vi "Loop_Overlord.vi"() -> ()   [LabVIEW 2017, in "Rotation_Overlord.lvlib"]
uses:
  Rotation_Overlord.lvlib
  _SHARE ALL/Global Share All/Global_STOP.vi
  ENUM_Overloard_Action.ctl
  ENUM_Overloard_State.ctl
  Arm/ENUM_SM_Rotate_Positions.ctl
  Arm/Arm.lvlib
  Arm/CLUSTER_CMD_SM_Lift_Rotate.ctl
  Claw Rotation/ENUM_SM_Rotate_Positions.ctl
  Claw Rotation/Claw_Rotation.lvlib
  Claw Rotation/CLUSTER_CMD_SM_Lift_Rotate.ctl
  Lift/ENUM_SM_Rotate_Positions.ctl
  Lift/Lift.lvlib
  Lift/CLUSTER_CMD_SM_Lift_Rotate.ctl
  Arm/Global_CMD.vi
  Claw Rotation/Global_CMD.vi
  Lift/Global_CMD.vi
  ENUM_Rotation_Positon.ctl
  CLUSTER_Rotation_CMD.ctl
  Global_CMD.vi
  Arm/ENUM_SM_State.ctl
  Claw Rotation/ENUM_SM_State.ctl
  Lift/ENUM_SM_State.ctl
  Arm/Global_SM Write_Data Out.vi
  Claw Rotation/Global_SM Write_Data Out.vi
  Lift/Global_SM Write_Data Out.vi
panel:
  out "Input DBL Data":dbl
  out "Output Bool Data":bool
  out "Output DBL Data":dbl
  out "OutputI INT Data":i32
  out "Cycle Time (S)":dbl format="%.3g"
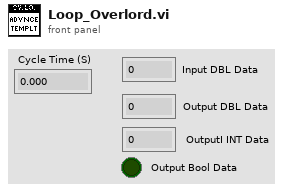
[diagram p1: front panel]
types:
  T1 = typedef "Lift.lvlib/ENUM_SM_State.ctl" = enum16{"Startup", "Idle", "Manual", "Position - Moving", "Position - Holding", "Shutdown"}
  T2 = typedef "Claw_Rotation.lvlib/ENUM_SM_State.ctl" = enum16{"Startup", "Idle", "Manual", "Position - Moving", "Position - Holding", "Shutdown"}
  T3 = typedef "Arm.lvlib/ENUM_SM_State.ctl" = enum16{"Startup", "Idle", "Manual", "Position - Moving", "Position - Holding", "Shutdown"}
  T4 = typedef "Rotation_Overlord.lvlib/CLUSTER_Rotation_CMD.ctl" = cluster{"Rotation Positon":T5, "Enable Rotation":bool}
  T5 = typedef "Rotation_Overlord.lvlib/ENUM_Rotation_Positon.ctl" = enum16{"Neutral", "Pickup", "Exchange", "Switch", "Scale", "Climb", "Manual"}
  T6 = typedef "Lift.lvlib/CLUSTER_CMD_SM_Lift_Rotate.ctl" = cluster{"Enable System":bool, "Rotate Position":T7, "Manual Velocity":dbl, "Manual Mode":bool}
  T7 = typedef "Lift.lvlib/ENUM_SM_Rotate_Positions.ctl" = enum16{"Neutral: 0", "Pickup: 0", "Exchange: 0", "Switch: 0", "Scale: 0", "Climb: 0"}
  T8 = typedef "Claw_Rotation.lvlib/CLUSTER_CMD_SM_Lift_Rotate.ctl" = cluster{"Enable System":bool, "Rotate Position":T9, "Manual Velocity":dbl, "Manual Mode":bool}
  T9 = typedef "Claw_Rotation.lvlib/ENUM_SM_Rotate_Positions.ctl" = enum16{"Neutral: 0", "Pickup: 0", "Exchange: 0", "Switch: 0", "Scale: 0", "Climb: 0"}
  T10 = typedef "Arm.lvlib/CLUSTER_CMD_SM_Lift_Rotate.ctl" = cluster{"Enable System":bool, "Rotate Position":T11, "Manual Velocity":dbl, "Manual Mode":bool}
  T11 = typedef "Arm.lvlib/ENUM_SM_Rotate_Positions.ctl" = enum16{"Neutral: 0", "Pickup: 0", "Exchange: 0", "Switch: 0", "Scale: 0", "Climb: 0"}
  T12 = typedef "Rotation_Overlord.lvlib/ENUM_Overloard_State.ctl" = enum16{"Startup", "Idle", "Neutral - Moving", "Neutral - Holding", "Pickup - Moving", "Pickup - Holding", "Exchange - Moving", "Exchange - Holding", "Switch - Moving", "Switch - Holding", "Scale - Moving", "Scale - Holding", "Climb - Moving", "Climb - Holding", "Manual", "Shutdown"}
  T13 = typedef "Rotation_Overlord.lvlib/ENUM_Overloard_Action.ctl" = enum16{"No Action", "Reset Time", "Disable All", "Disable Lift", "Disable Arm", "Disable Claw Rotation", "Set Neutral", "Set Pickup", "Set Exchange", "Set Switch", "Set Scale", "Set Climb", "Manual"}
  T14 = cluster{"State":T12, "Previous State":T12, "Current Time":timestamp, "Previous Time":timestamp, "Start Time":timestamp, "Target Time (ms)":u32, "Cycle Time(S)":dbl, "Arm CMD":T10, "Claw Rotation CMD":T8, "Lift CMD":T6, "Rotation CMD":T4, "Arm State":T3, "Claw Rotation State":T2, "Lift State":T1}
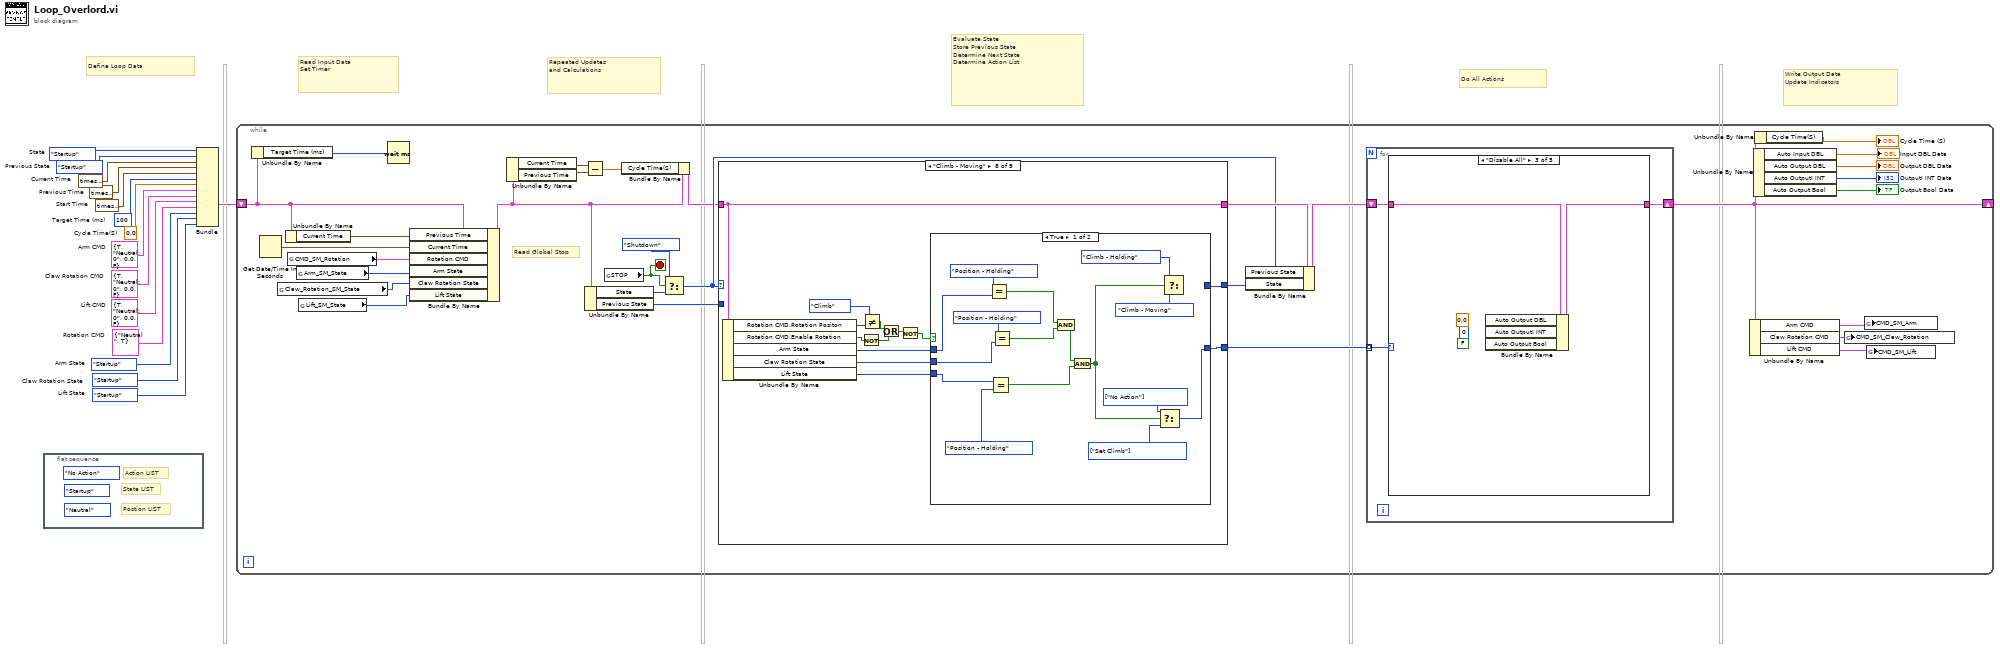
[diagram p0: block diagram]
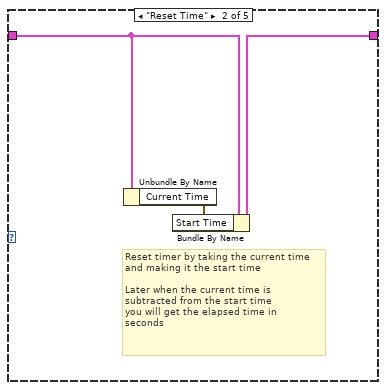
[diagram p3: hidden frame]
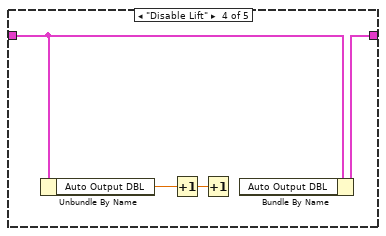
[diagram p4: hidden frame]
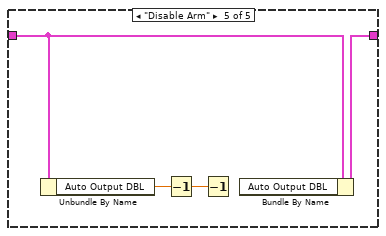
[diagram p5: hidden frame]
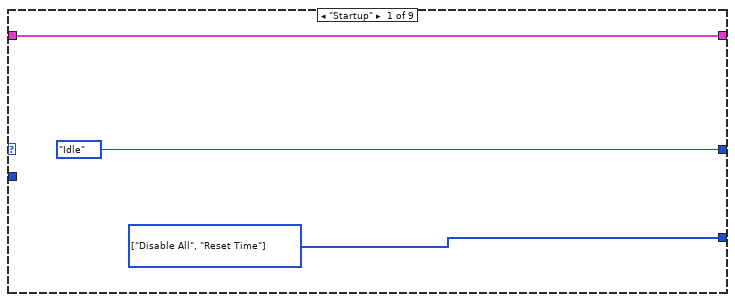
[diagram p6: hidden frame]
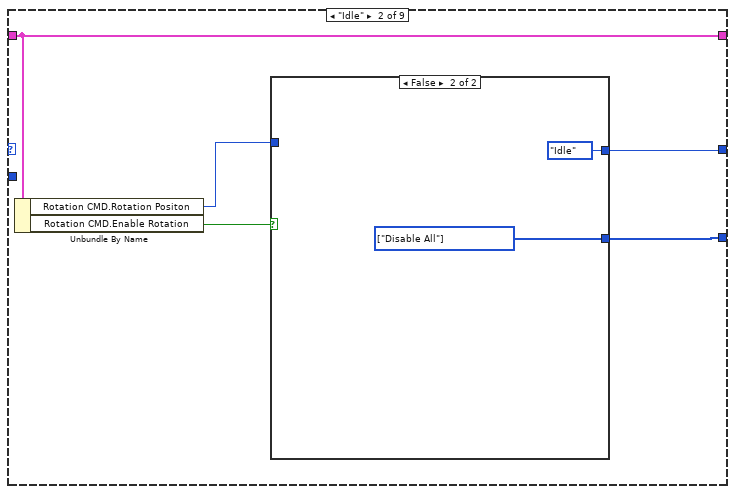
[diagram p7: hidden frame]
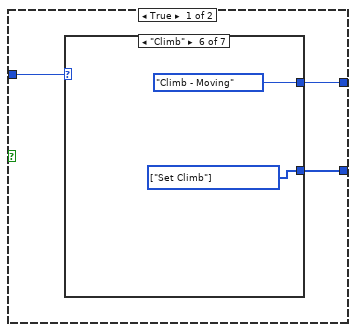
[diagram p8: hidden frame]
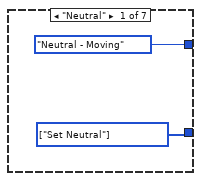
[diagram p9: hidden frame]
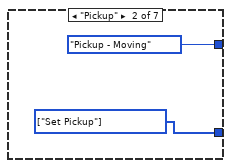
[diagram p10: hidden frame]
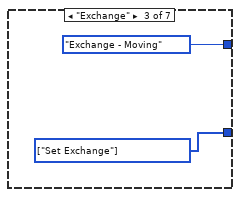
[diagram p11: hidden frame]
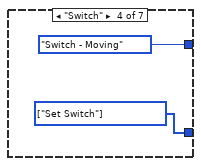
[diagram p12: hidden frame]
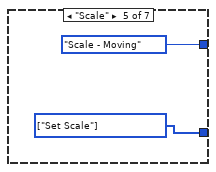
[diagram p13: hidden frame]
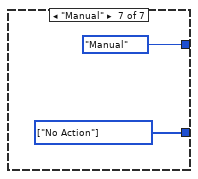
[diagram p14: hidden frame]
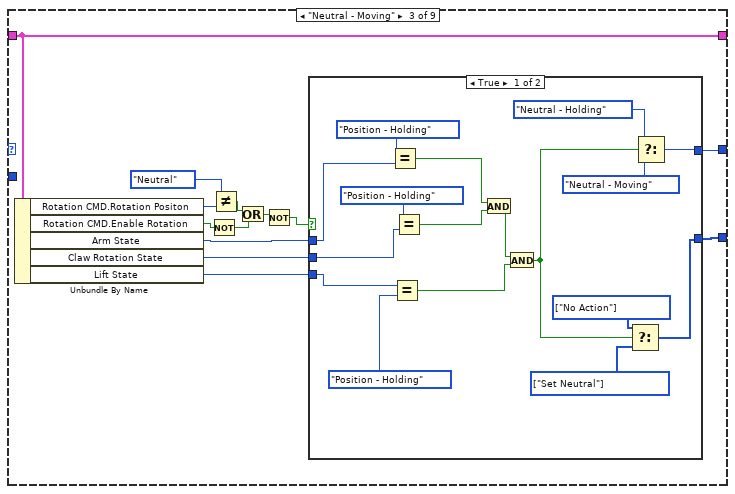
[diagram p15: hidden frame]
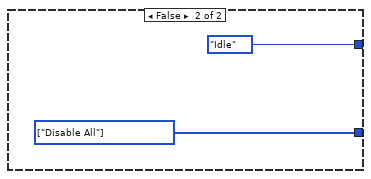
[diagram p16: hidden frame]
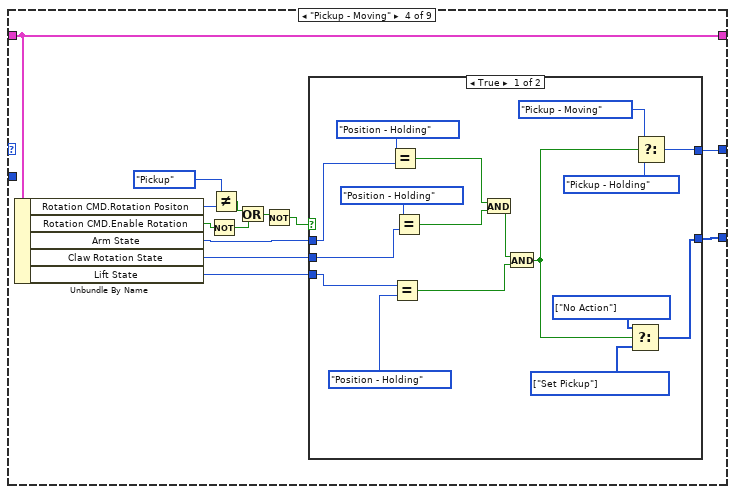
[diagram p17: hidden frame]
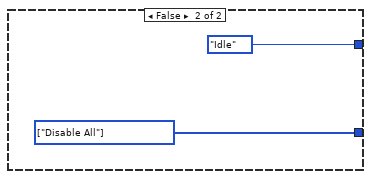
[diagram p18: hidden frame]
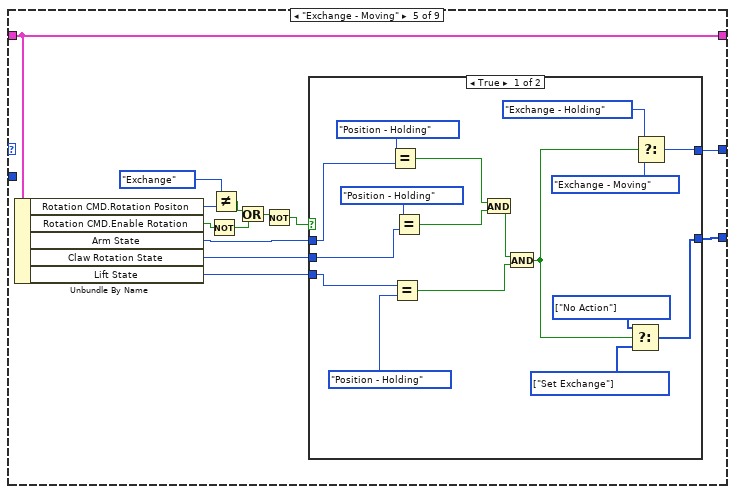
[diagram p19: hidden frame]
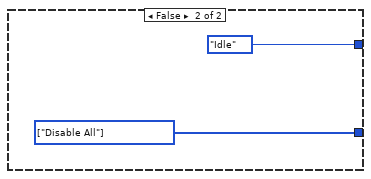
[diagram p20: hidden frame]
diagram:
  w1 = ENUM_SM_State."Startup"  # Lift State
  w2 = ENUM_SM_State."Startup"  # Claw Rotation State
  w3 = ENUM_SM_State."Startup"  # Arm State
  w4 = T4 {"Rotation Positon"=enum."Neutral", "Enable Rotation"=TRUE}  # Rotation CMD
  w5 = T6 {"Enable System"=TRUE, "Rotate Position"=enum."Neutral: 0", "Manual Velocity"=0.0, "Manual Mode"=FALSE}  # Lift CMD
  w6 = T8 {"Enable System"=TRUE, "Rotate Position"=enum."Neutral: 0", "Manual Velocity"=0.0, "Manual Mode"=FALSE}  # Claw Rotation CMD
  w7 = T10 {"Enable System"=TRUE, "Rotate Position"=enum."Neutral: 0", "Manual Velocity"=0.0, "Manual Mode"=FALSE}  # Arm CMD
  w8 = 0.0  # Cycle Time(S)
  w9 = ENUM_Overloard_State."Startup"  # Previous State
  w10 = timestamp(0 s since 1904-01-01)  # Previous Time
  w11 = u32 100  # Target Time (ms)
  w12 = timestamp(0 s since 1904-01-01)  # Start Time
  w13 = timestamp(0 s since 1904-01-01)  # Current Time
  w14 = ENUM_Overloard_State."Startup"  # State
  # "Define Loop Data"
  # "Repeated Updates\nand Calculations"
  # "Read Input Data\nSet Timer"
  # "Evaluate State\nStore Previous State\nDetermine Next State\nDetermine Action List"
  # "Do All Actions"
  # "Write Output Data\nUpdate Indicators"
  n1 = flat-sequence {
    frame #0 {
      (unwired) ENUM_Rotation_Positon."Neutral" ("Rotation Position")
      (unwired) ENUM_Overloard_State."Startup" ("State")
      (unwired) ENUM_Overloard_Action."No Action" ("Action")
      # "Postion LIST"
      # "State LIST"
      # "Action LIST"
    }
  }
  n2 = Bundle("State"=w14, "Previous State"=w9, "Current Time"=w13, "Previous Time"=w10, "Start Time"=w12, "Target Time (ms)"=w11, "Cycle Time(S)"=w8, "Arm CMD"=w7, "Claw Rotation CMD"=w6, "Lift CMD"=w5, "Rotation CMD"=w4, "Arm State"=w3, "Claw Rotation State"=w2, "Lift State"=w1) -> (w15:T14)  [unwired: 1 in]
  n3 = while {
    shift-right: [w32] -> _
    shift-left: w15 -> [w38]
    stop <- w21 stop-if-true
    # "Read Global Stop"
    n4 = Unbundle By Name(w38) -> ("Target Time (ms)"=w40:u32)
    n5 = Get Date/Time In Seconds() -> (seconds since 1Jan1904=w46:timestamp)
    n6 = global read "Global_SM Write_Data Out.vi" "Claw_Rotation_SM_State"() -> (w18:T2)
    n7 = Unbundle By Name(w38) -> ("Current Time"=w39:timestamp)
    n8 = global read "Global_CMD.vi" "CMD_SM_Rotation"() -> (w20:T4)
    n9 = global read "Global_SM Write_Data Out.vi" "Arm_SM_State"() -> (w19:T3)
    n10 = global read "Global_SM Write_Data Out.vi" "Lift_SM_State"() -> (w17:T1)
    n11 = Wait (ms)(milliseconds to wait=w40) -> ()  [unwired: 1 out]
    n12 = Bundle By Name(cluster=w38, "Previous Time"=w39, "Current Time"=w46, "Rotation CMD"=w20, "Arm State"=w19, "Claw Rotation State"=w18, "Lift State"=w17) -> (w28:T14)
    n13 = Unbundle By Name(w28) -> ("Current Time"=w29:timestamp, "Previous Time"=w30:timestamp)
    n14 = Subtract(x=w29, y=w30) -> (x-y=w26:dbl)
    n15 = Unbundle By Name(w28) -> ("State"=w41:T12, "Previous State"=w37:T12)
    n16 = global read "Global_STOP.vi" "STOP"() -> (w21:bool)
    n17 = Bundle By Name(cluster=w28, "Cycle Time(S)"=w26) -> (w27:T14)
    n18 = Select(t=ENUM_Overloard_State."Shutdown" ("State"), s=w21, f=w41) -> (s? t:f=w33:T12)
    n19 = case shown="\"Climb - Moving\"" w33 {
      tunnel: w27 -> [w66 w71 w103 w135 w167 w199 w230 w261 w282]
      tunnel: [w66 w71 w103 w135 w167 w199 w230 w261 w282] -> w44
      tunnel: [ENUM_Overloard_State."Idle" ("State") w67 w101 w133 w165 w197 w228 w259 ENUM_Overloard_State."Shutdown" ("State")] -> w43
      tunnel: w37 -> [_ _ _ _ _ _ _ _ _]
      tunnel: [w64 w69 w102 w134 w166 w198 w229 w260 w280] -> w16
      frame "Startup" {
        w64 = T13[] [enum."Disable All", enum."Reset Time"] items=["No Action", "Reset Time", "Disable All", "Disable Lift", "Disable Arm", "Disable Claw Rotation", "Set Neutral", "Set Pickup", "Set Exchange", "Set Switch", "Set Scale", "Set Climb", "Manual"] ("Actions")
      }
      frame "Idle" {
        n20 = Unbundle By Name(w71) -> ("Rotation CMD.Rotation Positon"=w68:T5, "Rotation CMD.Enable Rotation"=w70:bool)
        n21 = case shown="False" w70 {
          tunnel: [w72 w90] -> w69
          tunnel: w68 -> [w74 _]
          tunnel: [w73 ENUM_Overloard_State."Idle" ("State")] -> w67
          frame True {
            n22 = case shown="\"Climb\"" w74 {
              tunnel: [ENUM_Overloard_State."Neutral - Moving" ("State") ENUM_Overloard_State."Pickup - Moving" ("State") ENUM_Overloard_State."Exchange - Moving" ("State") ENUM_Overloard_State."Switch - Moving" ("State") ENUM_Overloard_State."Scale - Moving" ("State") ENUM_Overloard_State."Climb - Moving" ("State") ENUM_Overloard_State."Manual" ("State")] -> w73
              tunnel: [w75 w77 w79 w81 w83 w85 w87] -> w72
              frame "Neutral" {
                w75 = T13[] [enum."Set Neutral"] items=["No Action", "Reset Time", "Disable All", "Disable Lift", "Disable Arm", "Disable Claw Rotation", "Set Neutral", "Set Pickup", "Set Exchange", "Set Switch", "Set Scale", "Set Climb", "Manual"] ("Actions")
              }
              frame "Pickup" {
                w77 = T13[] [enum."Set Pickup"] items=["No Action", "Reset Time", "Disable All", "Disable Lift", "Disable Arm", "Disable Claw Rotation", "Set Neutral", "Set Pickup", "Set Exchange", "Set Switch", "Set Scale", "Set Climb", "Manual"] ("Actions")
              }
              frame "Exchange" {
                w79 = T13[] [enum."Set Exchange"] items=["No Action", "Reset Time", "Disable All", "Disable Lift", "Disable Arm", "Disable Claw Rotation", "Set Neutral", "Set Pickup", "Set Exchange", "Set Switch", "Set Scale", "Set Climb", "Manual"] ("Actions")
              }
              frame "Switch" {
                w81 = T13[] [enum."Set Switch"] items=["No Action", "Reset Time", "Disable All", "Disable Lift", "Disable Arm", "Disable Claw Rotation", "Set Neutral", "Set Pickup", "Set Exchange", "Set Switch", "Set Scale", "Set Climb", "Manual"] ("Actions")
              }
              frame "Scale" {
                w83 = T13[] [enum."Set Scale"] items=["No Action", "Reset Time", "Disable All", "Disable Lift", "Disable Arm", "Disable Claw Rotation", "Set Neutral", "Set Pickup", "Set Exchange", "Set Switch", "Set Scale", "Set Climb", "Manual"] ("Actions")
              }
              frame "Climb" {
                w85 = T13[] [enum."Set Climb"] items=["No Action", "Reset Time", "Disable All", "Disable Lift", "Disable Arm", "Disable Claw Rotation", "Set Neutral", "Set Pickup", "Set Exchange", "Set Switch", "Set Scale", "Set Climb", "Manual"] ("Actions")
              }
              frame "Manual" {
                w87 = T13[] [enum."No Action"] items=["No Action", "Reset Time", "Disable All", "Disable Lift", "Disable Arm", "Disable Claw Rotation", "Set Neutral", "Set Pickup", "Set Exchange", "Set Switch", "Set Scale", "Set Climb", "Manual"] ("Actions")
              }
            }
          }
          frame False {
            w90 = T13[] [enum."Disable All"] items=["No Action", "Reset Time", "Disable All", "Disable Lift", "Disable Arm", "Disable Claw Rotation", "Set Neutral", "Set Pickup", "Set Exchange", "Set Switch", "Set Scale", "Set Climb", "Manual"] ("Actions")
          }
        }
      }
      frame "Neutral - Moving" {
        n23 = Unbundle By Name(w103) -> ("Rotation CMD.Rotation Positon"=w100:T5, "Rotation CMD.Enable Rotation"=w98:bool, "Arm State"=w93:T3, "Claw Rotation State"=w92:T2, "Lift State"=w91:T1)
        n24 = Not(x=w98) -> (.not. x?=w96:bool)
        n25 = Not Equal?(x=ENUM_Rotation_Positon."Neutral", y=w100) -> (x != y?=w97:bool)
        n26 = Or(x=w97, y=w96) -> (x .or. y?=w95:bool)
        n27 = Not(x=w95) -> (.not. x?=w94:bool)
        n28 = case shown="True" w94 {
          tunnel: [w105 w122] -> w102
          tunnel: [w104 ENUM_Overloard_State."Idle" ("State")] -> w101
          tunnel: w93 -> [w120 _]
          tunnel: w92 -> [w119 _]
          tunnel: w91 -> [w118 _]
          frame True {
            w107 = T13[] [enum."Set Neutral"] items=["No Action", "Reset Time", "Disable All", "Disable Lift", "Disable Arm", "Disable Claw Rotation", "Set Neutral", "Set Pickup", "Set Exchange", "Set Switch", "Set Scale", "Set Climb", "Manual"] ("Actions")
            w106 = T13[] [enum."No Action"] items=["No Action", "Reset Time", "Disable All", "Disable Lift", "Disable Arm", "Disable Claw Rotation", "Set Neutral", "Set Pickup", "Set Exchange", "Set Switch", "Set Scale", "Set Climb", "Manual"] ("Actions")
            n29 = Equal?(x=ENUM_SM_State."Position - Holding", y=w120) -> (x = y?=w114:bool)
            n30 = Equal?(x=w118, y=ENUM_SM_State."Position - Holding") -> (x = y?=w111:bool)
            n31 = Equal?(x=ENUM_SM_State."Position - Holding", y=w119) -> (x = y?=w113:bool)
            n32 = And(x=w114, y=w113) -> (x .and. y?=w112:bool)
            n33 = And(x=w112, y=w111) -> (x .and. y?=w108:bool)
            n34 = Select(t=w106, s=w108, f=w107) -> (s? t:f=w105:T13[])
            n35 = Select(t=ENUM_Overloard_State."Neutral - Holding" ("State"), s=w108, f=ENUM_Overloard_State."Neutral - Moving" ("State")) -> (s? t:f=w104:T12)
          }
          frame False {
            w122 = T13[] [enum."Disable All"] items=["No Action", "Reset Time", "Disable All", "Disable Lift", "Disable Arm", "Disable Claw Rotation", "Set Neutral", "Set Pickup", "Set Exchange", "Set Switch", "Set Scale", "Set Climb", "Manual"] ("Actions")
          }
        }
      }
      frame "Pickup - Moving" {
        n36 = Unbundle By Name(w135) -> ("Rotation CMD.Rotation Positon"=w132:T5, "Rotation CMD.Enable Rotation"=w130:bool, "Arm State"=w125:T3, "Claw Rotation State"=w124:T2, "Lift State"=w123:T1)
        n37 = Not(x=w130) -> (.not. x?=w128:bool)
        n38 = Not Equal?(x=ENUM_Rotation_Positon."Pickup", y=w132) -> (x != y?=w129:bool)
        n39 = Or(x=w129, y=w128) -> (x .or. y?=w127:bool)
        n40 = Not(x=w127) -> (.not. x?=w126:bool)
        n41 = case shown="True" w126 {
          tunnel: [w137 w154] -> w134
          tunnel: [w136 ENUM_Overloard_State."Idle" ("State")] -> w133
          tunnel: w125 -> [w152 _]
          tunnel: w124 -> [w151 _]
          tunnel: w123 -> [w150 _]
          frame True {
            w139 = T13[] [enum."Set Pickup"] items=["No Action", "Reset Time", "Disable All", "Disable Lift", "Disable Arm", "Disable Claw Rotation", "Set Neutral", "Set Pickup", "Set Exchange", "Set Switch", "Set Scale", "Set Climb", "Manual"] ("Actions")
            w138 = T13[] [enum."No Action"] items=["No Action", "Reset Time", "Disable All", "Disable Lift", "Disable Arm", "Disable Claw Rotation", "Set Neutral", "Set Pickup", "Set Exchange", "Set Switch", "Set Scale", "Set Climb", "Manual"] ("Actions")
            n42 = Equal?(x=ENUM_SM_State."Position - Holding", y=w152) -> (x = y?=w146:bool)
            n43 = Equal?(x=w150, y=ENUM_SM_State."Position - Holding") -> (x = y?=w143:bool)
            n44 = Equal?(x=ENUM_SM_State."Position - Holding", y=w151) -> (x = y?=w145:bool)
            n45 = And(x=w146, y=w145) -> (x .and. y?=w144:bool)
            n46 = And(x=w144, y=w143) -> (x .and. y?=w140:bool)
            n47 = Select(t=w138, s=w140, f=w139) -> (s? t:f=w137:T13[])
            n48 = Select(t=ENUM_Overloard_State."Pickup - Moving" ("State"), s=w140, f=ENUM_Overloard_State."Pickup - Holding" ("State")) -> (s? t:f=w136:T12)
          }
          frame False {
            w154 = T13[] [enum."Disable All"] items=["No Action", "Reset Time", "Disable All", "Disable Lift", "Disable Arm", "Disable Claw Rotation", "Set Neutral", "Set Pickup", "Set Exchange", "Set Switch", "Set Scale", "Set Climb", "Manual"] ("Actions")
          }
        }
      }
      frame "Exchange - Moving" {
        n49 = Unbundle By Name(w167) -> ("Rotation CMD.Rotation Positon"=w164:T5, "Rotation CMD.Enable Rotation"=w162:bool, "Arm State"=w157:T3, "Claw Rotation State"=w156:T2, "Lift State"=w155:T1)
        n50 = Not(x=w162) -> (.not. x?=w160:bool)
        n51 = Not Equal?(x=ENUM_Rotation_Positon."Exchange", y=w164) -> (x != y?=w161:bool)
        n52 = Or(x=w161, y=w160) -> (x .or. y?=w159:bool)
        n53 = Not(x=w159) -> (.not. x?=w158:bool)
        n54 = case shown="True" w158 {
          tunnel: [w169 w186] -> w166
          tunnel: [w168 ENUM_Overloard_State."Idle" ("State")] -> w165
          tunnel: w157 -> [w184 _]
          tunnel: w156 -> [w183 _]
          tunnel: w155 -> [w182 _]
          frame True {
            w171 = T13[] [enum."Set Exchange"] items=["No Action", "Reset Time", "Disable All", "Disable Lift", "Disable Arm", "Disable Claw Rotation", "Set Neutral", "Set Pickup", "Set Exchange", "Set Switch", "Set Scale", "Set Climb", "Manual"] ("Actions")
            w170 = T13[] [enum."No Action"] items=["No Action", "Reset Time", "Disable All", "Disable Lift", "Disable Arm", "Disable Claw Rotation", "Set Neutral", "Set Pickup", "Set Exchange", "Set Switch", "Set Scale", "Set Climb", "Manual"] ("Actions")
            n55 = Equal?(x=ENUM_SM_State."Position - Holding", y=w184) -> (x = y?=w178:bool)
            n56 = Equal?(x=w182, y=ENUM_SM_State."Position - Holding") -> (x = y?=w175:bool)
            n57 = Equal?(x=ENUM_SM_State."Position - Holding", y=w183) -> (x = y?=w177:bool)
            n58 = And(x=w178, y=w177) -> (x .and. y?=w176:bool)
            n59 = And(x=w176, y=w175) -> (x .and. y?=w172:bool)
            n60 = Select(t=w170, s=w172, f=w171) -> (s? t:f=w169:T13[])
            n61 = Select(t=ENUM_Overloard_State."Exchange - Holding" ("State"), s=w172, f=ENUM_Overloard_State."Exchange - Moving" ("State")) -> (s? t:f=w168:T12)
          }
          frame False {
            w186 = T13[] [enum."Disable All"] items=["No Action", "Reset Time", "Disable All", "Disable Lift", "Disable Arm", "Disable Claw Rotation", "Set Neutral", "Set Pickup", "Set Exchange", "Set Switch", "Set Scale", "Set Climb", "Manual"] ("Actions")
          }
        }
      }
      frame "Switch - Moving" {
        n62 = Unbundle By Name(w199) -> ("Rotation CMD.Rotation Positon"=w196:T5, "Rotation CMD.Enable Rotation"=w194:bool, "Arm State"=w189:T3, "Claw Rotation State"=w188:T2, "Lift State"=w187:T1)
        n63 = Not(x=w194) -> (.not. x?=w192:bool)
        n64 = Not Equal?(x=ENUM_Rotation_Positon."Switch", y=w196) -> (x != y?=w193:bool)
        n65 = Or(x=w193, y=w192) -> (x .or. y?=w191:bool)
        n66 = Not(x=w191) -> (.not. x?=w190:bool)
        n67 = case shown="True" w190 {
          tunnel: [w200 w217] -> w198
          tunnel: [_ ENUM_Overloard_State."Idle" ("State")] -> w197
          tunnel: w189 -> [w215 _]
          tunnel: w188 -> [w214 _]
          tunnel: w187 -> [w213 _]
          frame True {
            w202 = T13[] [enum."Set Switch"] items=["No Action", "Reset Time", "Disable All", "Disable Lift", "Disable Arm", "Disable Claw Rotation", "Set Neutral", "Set Pickup", "Set Exchange", "Set Switch", "Set Scale", "Set Climb", "Manual"] ("Actions")
            w201 = T13[] [enum."No Action"] items=["No Action", "Reset Time", "Disable All", "Disable Lift", "Disable Arm", "Disable Claw Rotation", "Set Neutral", "Set Pickup", "Set Exchange", "Set Switch", "Set Scale", "Set Climb", "Manual"] ("Actions")
            n68 = Equal?(x=ENUM_SM_State."Position - Holding", y=w215) -> (x = y?=w209:bool)
            n69 = Equal?(x=w213, y=ENUM_SM_State."Position - Holding") -> (x = y?=w206:bool)
            n70 = Equal?(x=ENUM_SM_State."Position - Holding", y=w214) -> (x = y?=w208:bool)
            n71 = And(x=w209, y=w208) -> (x .and. y?=w207:bool)
            n72 = And(x=w207, y=w206) -> (x .and. y?=w203:bool)
            n73 = Select(t=w201, s=w203, f=w202) -> (s? t:f=w200:T13[])
            n74 = Select(t=ENUM_Overloard_State."Switch - Holding" ("State"), s=w203, f=ENUM_Overloard_State."Switch - Moving" ("State")) -> ()  [unwired: 1 out]
          }
          frame False {
            w217 = T13[] [enum."Disable All"] items=["No Action", "Reset Time", "Disable All", "Disable Lift", "Disable Arm", "Disable Claw Rotation", "Set Neutral", "Set Pickup", "Set Exchange", "Set Switch", "Set Scale", "Set Climb", "Manual"] ("Actions")
          }
        }
      }
      frame "Scale - Moving" {
        n75 = Unbundle By Name(w230) -> ("Rotation CMD.Rotation Positon"=w227:T5, "Rotation CMD.Enable Rotation"=w225:bool, "Arm State"=w220:T3, "Claw Rotation State"=w219:T2, "Lift State"=w218:T1)
        n76 = Not(x=w225) -> (.not. x?=w223:bool)
        n77 = Not Equal?(x=ENUM_Rotation_Positon."Scale", y=w227) -> (x != y?=w224:bool)
        n78 = Or(x=w224, y=w223) -> (x .or. y?=w222:bool)
        n79 = Not(x=w222) -> (.not. x?=w221:bool)
        n80 = case shown="True" w221 {
          tunnel: [w231 w248] -> w229
          tunnel: [_ ENUM_Overloard_State."Idle" ("State")] -> w228
          tunnel: w220 -> [w246 _]
          tunnel: w219 -> [w245 _]
          tunnel: w218 -> [w244 _]
          frame True {
            w233 = T13[] [enum."Set Scale"] items=["No Action", "Reset Time", "Disable All", "Disable Lift", "Disable Arm", "Disable Claw Rotation", "Set Neutral", "Set Pickup", "Set Exchange", "Set Switch", "Set Scale", "Set Climb", "Manual"] ("Actions")
            w232 = T13[] [enum."No Action"] items=["No Action", "Reset Time", "Disable All", "Disable Lift", "Disable Arm", "Disable Claw Rotation", "Set Neutral", "Set Pickup", "Set Exchange", "Set Switch", "Set Scale", "Set Climb", "Manual"] ("Actions")
            n81 = Equal?(x=ENUM_SM_State."Position - Holding", y=w246) -> (x = y?=w240:bool)
            n82 = Equal?(x=w244, y=ENUM_SM_State."Position - Holding") -> (x = y?=w237:bool)
            n83 = Equal?(x=ENUM_SM_State."Position - Holding", y=w245) -> (x = y?=w239:bool)
            n84 = And(x=w240, y=w239) -> (x .and. y?=w238:bool)
            n85 = And(x=w238, y=w237) -> (x .and. y?=w234:bool)
            n86 = Select(t=w232, s=w234, f=w233) -> (s? t:f=w231:T13[])
            n87 = Select(t=ENUM_Overloard_State."Scale - Holding" ("State"), s=w234, f=ENUM_Overloard_State."Scale - Moving" ("State")) -> ()  [unwired: 1 out]
          }
          frame False {
            w248 = T13[] [enum."Disable All"] items=["No Action", "Reset Time", "Disable All", "Disable Lift", "Disable Arm", "Disable Claw Rotation", "Set Neutral", "Set Pickup", "Set Exchange", "Set Switch", "Set Scale", "Set Climb", "Manual"] ("Actions")
          }
        }
      }
      frame "Climb - Moving" {
        n88 = Unbundle By Name(w261) -> ("Rotation CMD.Rotation Positon"=w258:T5, "Rotation CMD.Enable Rotation"=w256:bool, "Arm State"=w251:T3, "Claw Rotation State"=w250:T2, "Lift State"=w249:T1)
        n89 = Not(x=w256) -> (.not. x?=w254:bool)
        n90 = Not Equal?(x=ENUM_Rotation_Positon."Climb", y=w258) -> (x != y?=w255:bool)
        n91 = Or(x=w255, y=w254) -> (x .or. y?=w253:bool)
        n92 = Not(x=w253) -> (.not. x?=w252:bool)
        n93 = case shown="True" w252 {
          tunnel: [w262 w279] -> w260
          tunnel: [_ ENUM_Overloard_State."Idle" ("State")] -> w259
          tunnel: w251 -> [w277 _]
          tunnel: w250 -> [w276 _]
          tunnel: w249 -> [w275 _]
          frame True {
            w264 = T13[] [enum."Set Climb"] items=["No Action", "Reset Time", "Disable All", "Disable Lift", "Disable Arm", "Disable Claw Rotation", "Set Neutral", "Set Pickup", "Set Exchange", "Set Switch", "Set Scale", "Set Climb", "Manual"] ("Actions")
            w263 = T13[] [enum."No Action"] items=["No Action", "Reset Time", "Disable All", "Disable Lift", "Disable Arm", "Disable Claw Rotation", "Set Neutral", "Set Pickup", "Set Exchange", "Set Switch", "Set Scale", "Set Climb", "Manual"] ("Actions")
            n94 = Equal?(x=ENUM_SM_State."Position - Holding", y=w277) -> (x = y?=w271:bool)
            n95 = Equal?(x=w275, y=ENUM_SM_State."Position - Holding") -> (x = y?=w268:bool)
            n96 = Equal?(x=ENUM_SM_State."Position - Holding", y=w276) -> (x = y?=w270:bool)
            n97 = And(x=w271, y=w270) -> (x .and. y?=w269:bool)
            n98 = And(x=w269, y=w268) -> (x .and. y?=w265:bool)
            n99 = Select(t=w263, s=w265, f=w264) -> (s? t:f=w262:T13[])
            n100 = Select(t=ENUM_Overloard_State."Climb - Holding" ("State"), s=w265, f=ENUM_Overloard_State."Climb - Moving" ("State")) -> ()  [unwired: 1 out]
          }
          frame False {
            w279 = T13[] [enum."Disable All"] items=["No Action", "Reset Time", "Disable All", "Disable Lift", "Disable Arm", "Disable Claw Rotation", "Set Neutral", "Set Pickup", "Set Exchange", "Set Switch", "Set Scale", "Set Climb", "Manual"] ("Actions")
          }
        }
      }
      frame "Shutdown" {
        w280 = T13[] [enum."Disable All"] items=["No Action", "Reset Time", "Disable All", "Disable Lift", "Disable Arm", "Disable Claw Rotation", "Set Neutral", "Set Pickup", "Set Exchange", "Set Switch", "Set Scale", "Set Climb", "Manual"] ("Actions")
      }
    }
    n101 = Bundle By Name(cluster=w44, "Previous State"=w33, "State"=w43) -> (w45:T14)
    n102 = for {
      shift-right: [w49] -> w32
      shift-left: w45 -> [w48]
      tunnel: w16 -> [w47] mode=indexing
      n103 = case shown="\"Disable All\"" w47 {
        tunnel: w48 -> [w50 w53 w55 w58 w62]
        tunnel: [w50 w52 w54 w57 w61] -> w49
        frame "No Action" {
        }
        frame "Reset Time" {
          # "Reset timer by taking the current time\nand making it the start time\n\nLater when the current time is \nsubtracted from the start time\nyou will get the elapsed time in \nseconds"
          n104 = Unbundle By Name(w53) -> ("Current Time"=w51:timestamp)
          n105 = Bundle By Name(cluster=w53, "Start Time"=w51) -> (w52:T14)
        }
        frame "Disable All" {
          (unwired) FALSE ("Output Bool")
          (unwired) 0 ("OutputI INT")
          (unwired) 0.0 ("FG Write Value")
          n106 = Bundle By Name(cluster=w55) -> (w54:T14)  [unwired: 3 in]
        }
        frame "Disable Lift" {
          n107 = Unbundle By Name(w58) -> ("Auto Output DBL"=w59:dbl)
          n108 = Increment(x=w59) -> (x+1=w56:dbl)
          n109 = Increment(x=w56) -> ()  [unwired: 1 out]
          n110 = Bundle By Name(cluster=w58) -> (w57:T14)  [unwired: 1 in]
        }
        frame "Disable Arm" {
          n111 = Unbundle By Name(w62) -> ("Auto Output DBL"=w63:dbl)
          n112 = Decrement(x=w63) -> (x-1=w60:dbl)
          n113 = Decrement(x=w60) -> ()  [unwired: 1 out]
          n114 = Bundle By Name(cluster=w62) -> (w61:T14)  [unwired: 1 in]
        }
      }
    }
    n115 = Unbundle By Name(w32) -> ("Arm CMD"=w24:T10, "Claw Rotation CMD"=w23:T8, "Lift CMD"=w22:T6)
    n116 = Unbundle By Name(w32) -> ("Auto Input DBL"=→"Input DBL Data":dbl, "Auto Output DBL"=→"Output DBL Data":dbl, "Auto OutputI INT"=→"OutputI INT Data":i32, "Auto Output Bool"=→"Output Bool Data":bool)
    n117 = Unbundle By Name(w32) -> ("Cycle Time(S)"=→"Cycle Time (S)":dbl)
    n118 = global write "Global_CMD.vi" "CMD_SM_Claw_Rotation"(w23) -> ()
    n119 = global write "Global_CMD.vi" "CMD_SM_Arm"(w24) -> ()
    n120 = global write "Global_CMD.vi" "CMD_SM_Lift"(w22) -> ()
  }
